vi "Test Resample.vi"() -> ()   [LabVIEW 2013, in "Data Log Fetcher.lvlib"]
uses:
  Data Log Fetcher.lvlib
panel:
  in  "Duration (s)":i32=3
  in  "Irregular Data":dbl[][](array[numeric])=[[0.0, 1.0, 1.5], [0.0, 2.0, 3.0]]
  out "Regular Data":dbl[][](array[numeric])
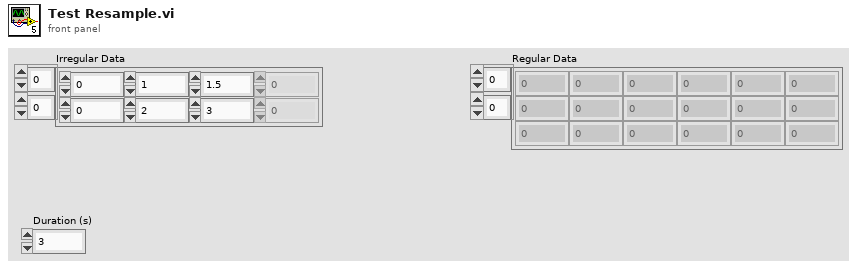
[diagram p1: front panel]
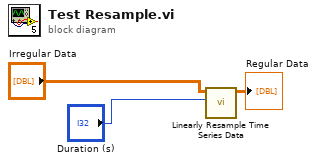
[diagram p0: block diagram]
diagram:
  n1 = call "Linearly Resample Time Series Data.vi"("Duration (s)"="Duration (s)", "Irregular Data"="Irregular Data") -> ("Regular Data"=→"Regular Data":dbl[][])  [unwired: 9 in]
